vi "Parse Button Label.vi"(0 "Label.Text":string) -> (14 "Stage Label":string, 15 "Increase?":bool=TRUE, 16 "Big Step?":bool)   [LabVIEW 2020]
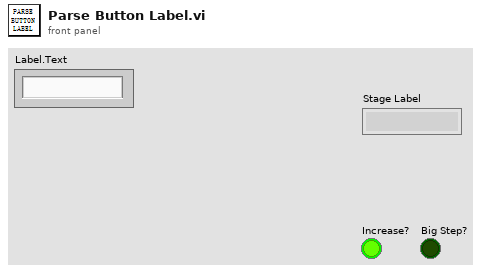
[diagram p1: front panel]
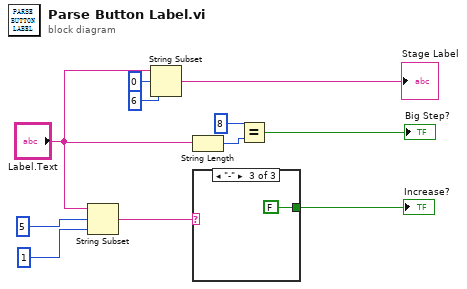
[diagram p0: block diagram]
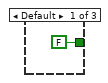
[diagram p2: hidden frame]
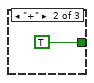
[diagram p3: hidden frame]
diagram:
  n1 = String Subset(string="Label.Text", offset (0)=5, length (rest)=1 ("length (rest)")) -> (substring=w9:string)
  n2 = String Subset(string="Label.Text", offset (0)=0, length (rest)=6 ("length (rest)")) -> (substring=→"Stage Label":string)
  n3 = String Length(string="Label.Text") -> (length=w3:i32)
  n4 = case shown="\"-\"" w9 {
    tunnel: [FALSE ("Increase?") TRUE ("Increase?") FALSE ("Increase?")] -> w8
    frame Default {
    }
    frame "+" {
    }
    frame "-" {
    }
  }
  "Increase?" <- w8
  n5 = Equal?(x=8, y=w3) -> (x = y?=→"Big Step?":bool)
